vi "Session.vi"() -> ()   [LabVIEW 2017]
uses:
  Control/Damping.ctl
  Global.vi
panel:
  in  "Type":enum16{"Mini45", "Joystick", "Simulation"}(ring)=enum."Simulation"
  out "Waveform Chart":dbl(graph)
  out "Reward":dbl(graph)
  out "Damping":T1={"Cx"=0.5493061443340549, "Cy"=0.5493061443340549, "Cz"=inf}
  in  "DDA":bool=TRUE
  out "error out":errorcluster
  in  "Stop":bool
  in  "error in":errorcluster
  in  "Exit":bool
  in  "Start":bool
  in  "ADL":u16(ring)=2 items=["None", "Book", "Pitcher", "Laptop", "Gear"]
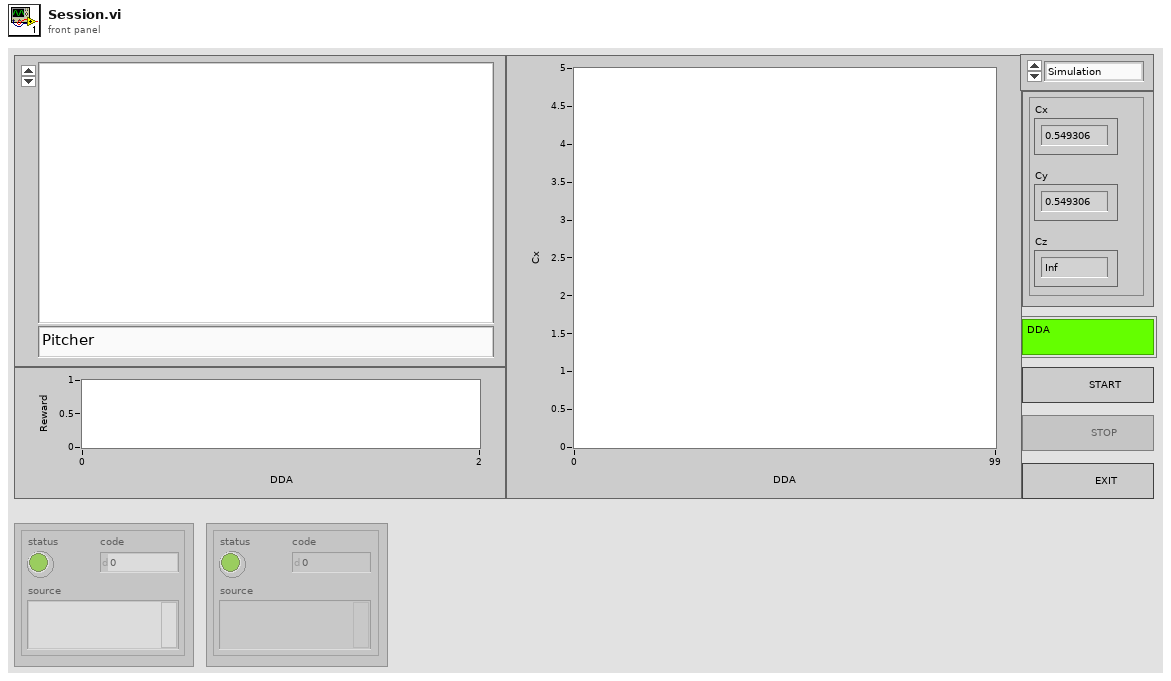
[diagram p1: front panel]
types:
  T1 = typedef "Damping.ctl" = cluster{"Cx":dbl, "Cy":dbl, "Cz":dbl}
  T2 = enum8{"Enabled", "Disabled", "Disabled and Grayed Out"}
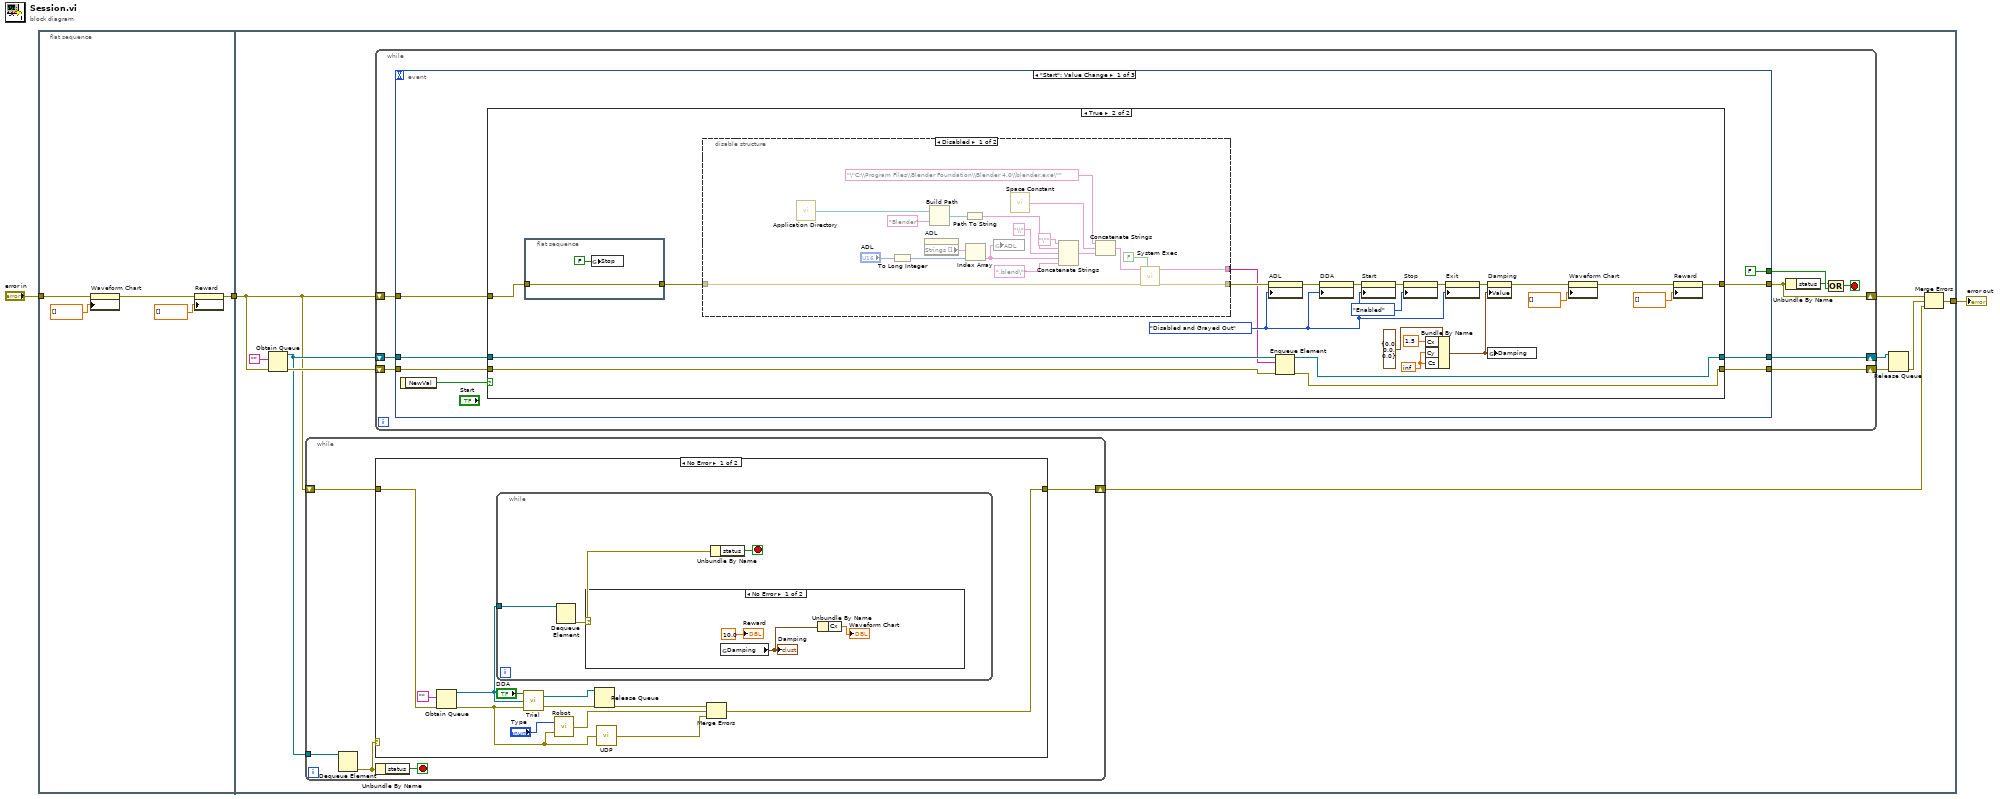
[diagram p0: block diagram]
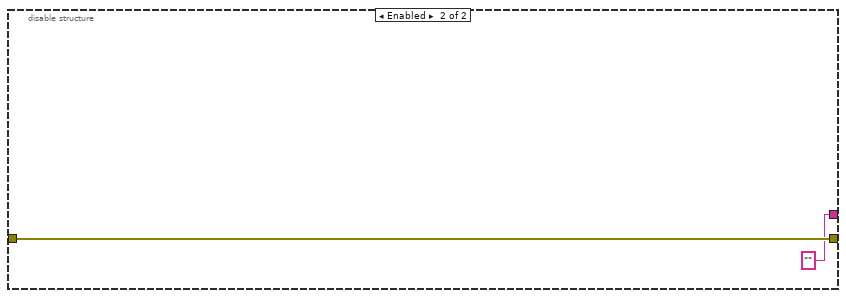
[diagram p3: hidden frame]
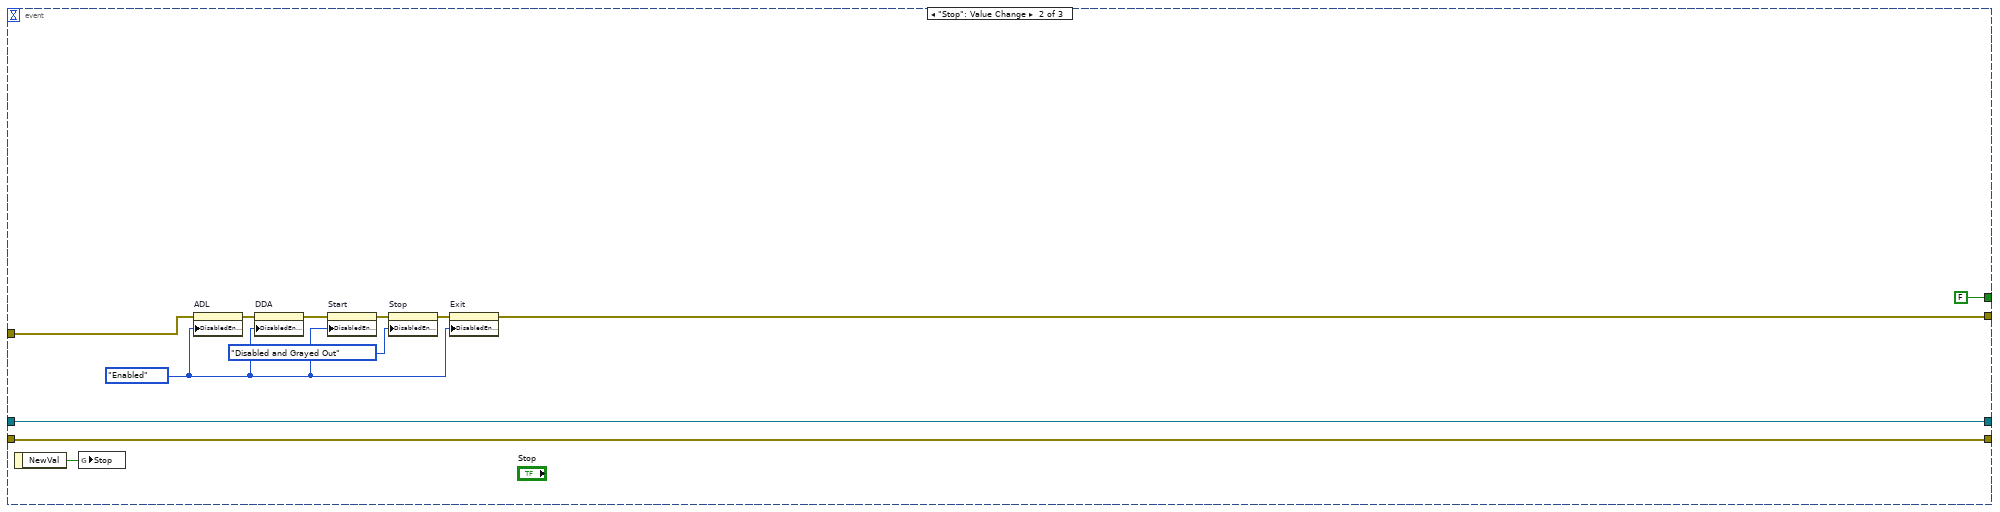
[diagram p4: hidden frame]
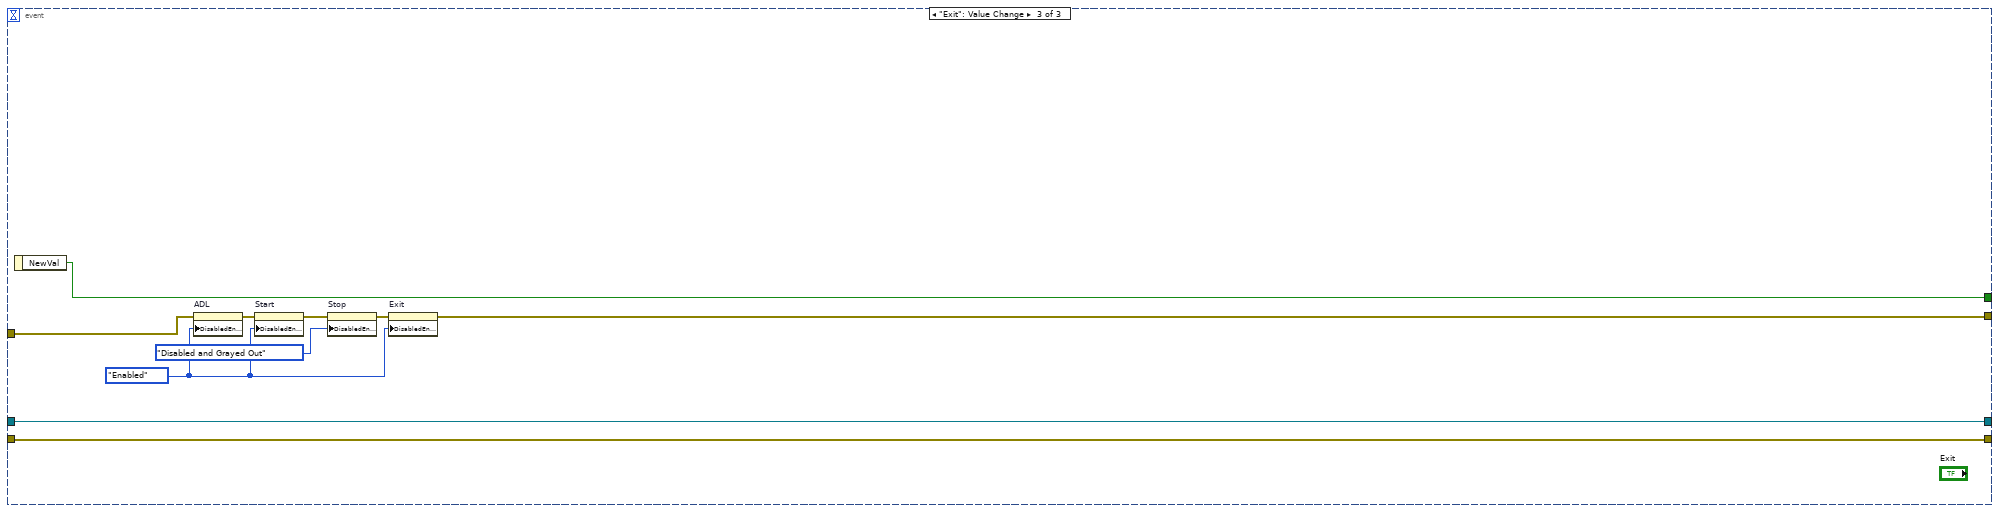
[diagram p5: hidden frame]
diagram:
  n1 = flat-sequence {
    tunnel: "error in" -> [w6]
    tunnel: [w4] -> w1
    tunnel: [w11] -> w3
    tunnel: w1 -> [w9]
    frame #0 {
      n2 = property on="Waveform Chart" class="WFChart (strict)"(error in=w6, "History Data"=dbl[] []) -> (error out=w5:errorcluster)  [unwired: 1 in, 1 out]
      n3 = property on="Reward" class="WFChart (strict)"(error in=w5, "History Data"=dbl[] []) -> (error out=w4:errorcluster)  [unwired: 1 in, 1 out]
    }
    frame #1 {
      n4 = Obtain Queue(element data type="", error in (no error)=w9) -> (queue out=w14:refnum<queue>, error out=w17:errorcluster)  [unwired: 3 in, 1 out]
      n5 = while {
        tunnel: w14 -> [w112]
        shift-right: [w109] -> w10
        shift-left: w9 -> [w108]
        stop <- w110 stop-if-true
        n6 = Dequeue Element(queue=w112) -> (error out=w111:errorcluster)  [unwired: 2 in, 3 out]
        n7 = case shown="No Error" w111 {
          tunnel: [w123 w131] -> w109
          tunnel: w108 -> [w122 w131]
          frame No Error {
            n8 = Obtain Queue(element data type="", error in (no error)=w122) -> (queue out=w116:refnum<queue>, error out=w115:errorcluster)  [unwired: 3 in, 1 out]
            n9 = while {
              tunnel: w116 -> [w126]
              stop <- w125 stop-if-true
              n10 = Dequeue Element(queue=w126) -> (error out=w127:errorcluster)  [unwired: 2 in, 3 out]
              n11 = case shown="No Error" w127 {
                frame No Error {
                  n12 = global read "Global.vi" "Damping"() -> (w130:T1)
                  "Damping" <- w130
                  n13 = Unbundle By Name(w130) -> ("Cx"=→"Waveform Chart":dbl)
                  "Reward" <- 10.0 ("Reward")
                }
                frame Error {
                }
              }
              n14 = Unbundle By Name(w127) -> ("status"=w125:bool)
            }
            n15 = call "Trial.vi"("error in (no error)"=w115, "queue in"=w116, "DDA"="DDA") -> ("error out"=w114:errorcluster, "queue out"=w113:refnum<queue>)
            n16 = call "Robot.vi"("error in"=w115, "Type"="Type") -> ("error out"=w119:errorcluster)
            n17 = Release Queue(queue=w113, error in (no error)=w114) -> (error out=w120:errorcluster)  [unwired: 1 in, 2 out]
            n18 = call "UDP.vi"("error in (no error)"=w115) -> ("error out"=w124:errorcluster)
            n19 = Merge Errors(w120, w119, w124) -> (w123:errorcluster)
          }
          frame Error {
          }
        }
        n20 = Unbundle By Name(w111) -> ("status"=w110:bool)
      }
      n21 = while {
        shift-right: [w26] -> w13
        shift-left: w9 -> [w27]
        shift-right: [w19] -> w15
        shift-left: w17 -> [w21]
        shift-right: [w20] -> w16
        shift-left: w14 -> [w22]
        stop <- w23 stop-if-true
        n22 = event shown="[0] \"Start\": Value Change" {
          selector: _ -> [_ _ _]
          dyn-events: _ -> [_ _ _]
          timeout: _ -> [_ _ _]
          tunnel: [w34 w93 w100] -> w26
          tunnel: w27 -> [w33 w86 w104]
          tunnel: [FALSE ("Stop") FALSE ("NewVal") w107] -> w25
          tunnel: w22 -> [w31 w94 w106]
          tunnel: w21 -> [w30 w95 w105]
          tunnel: [w29 w94 w106] -> w20
          tunnel: [w28 w95 w105] -> w19
          event "Start": Value Change {
            n23 = event-data() -> ("NewVal"=w35:bool)  [unwired: 1 in]
            n24 = case shown="True" w35 {
              tunnel: [w38 w45] -> w34
              tunnel: w33 -> [w38 w51]
              tunnel: w31 -> [w36 w62]
              tunnel: w30 -> [w37 w61]
              tunnel: [w36 w60] -> w29
              tunnel: [w37 w59] -> w28
              frame False {
              }
              frame True {
                w39 = inf
                w53 = T2."Disabled and Grayed Out" ("Disabled")
                n25 = flat-sequence {
                  tunnel: [w84] -> w49
                  tunnel: w51 -> [w84]
                  frame #0 {
                    n26 = global write "Global.vi" "Stop"(FALSE ("Stop")) -> ()
                  }
                }
                n27 = disable-structure shown="Disabled" {
                  disable-tunnel: [w69 w83] -> w58
                  disable-tunnel: w49 -> [w64 w83]
                  disable-tunnel: [w63 "" ("standard output")] -> w41
                  frame Disabled {
                    n28 = call <vilib>:"Application Directory.vi"() -> ("Application Directory"=w79:path)
                    n29 = To Long Integer(number="ADL") -> (32bit integer=w68:i32)
                    n30 = property on="ADL" class="Ring (strict)"() -> ("Strings []"=w81:string[])  [unwired: 2 in, 2 out]
                    n31 = Build Path(base path=w79, name or relative path="Blender") -> (appended path=w77:path)
                    n32 = Path To String(path=w77) -> (string=w76:string)
                    n33 = Index Array(array=w81, index=w68) -> (element=w67:string)
                    n34 = global write "Global.vi" "ADL"(w67) -> ()
                    n35 = call <vilib>:"Space Constant.vi"() -> ("String"=w72:string)
                    n36 = Concatenate Strings("\"" ("string"), w76, "\\" ("string"), w67, ".blend\"" ("string")) -> (w71:string)
                    n37 = Concatenate Strings("\"C:\\Program Files\\Blender Foundation\\Blender 4.0\\blender.exe\"" ("Blender Path"), w72, w71) -> (w70:string)
                    n38 = call <vilib>:"System Exec.vi"("wait until completion? (T)"=FALSE, "error in (no error)"=w64, "command line"=w70) -> ("error out"=w69:errorcluster, "standard output"=w63:string)  [unwired: 5 in, 2 out]
                  }
                  frame Enabled {
                  }
                }
                n39 = property on="ADL" class="Ring (strict)"(error in=w58, "DisabledEnum"=w53) -> (error out=w52:errorcluster)  [unwired: 1 in, 1 out]
                n40 = Enqueue Element(queue=w62, element=w41, error in (no error)=w61) -> (queue out=w60:refnum<queue>, error out=w59:errorcluster)  [unwired: 1 in, 1 out]
                n41 = property on="DDA" class="Bool (strict)"(error in=w52, "DisabledEnum"=w53) -> (error out=w54:errorcluster)  [unwired: 1 in, 1 out]
                n42 = property on="Start" class="Bool"(error in=w54, "DisabledEnum"=w53) -> (error out=w57:errorcluster)  [unwired: 1 in, 1 out]
                n43 = property on="Stop" class="Bool"(error in=w57, "DisabledEnum"=T2."Enabled" ("Disabled")) -> (error out=w56:errorcluster)  [unwired: 1 in, 1 out]
                n44 = Bundle By Name(cluster=T1 {"Cx"=0.0, "Cy"=0.0, "Cz"=0.0} ("State"), "Cx"=1.5, "Cy"=w39, "Cz"=w39) -> (w48:T1)
                n45 = property on="Exit" class="Bool"(error in=w56, "DisabledEnum"=w53) -> (error out=w47:errorcluster)  [unwired: 1 in, 1 out]
                n46 = property on="Damping" class="Clust (strict)"(error in=w47, "Value"=w48) -> (error out=w44:errorcluster)  [unwired: 1 in, 1 out]
                n47 = global write "Global.vi" "Damping"(w48) -> ()
                n48 = property on="Waveform Chart" class="WFChart (strict)"(error in=w44, "History Data"=dbl[] []) -> (error out=w43:errorcluster)  [unwired: 1 in, 1 out]
                n49 = property on="Reward" class="WFChart (strict)"(error in=w43, "History Data"=dbl[] []) -> (error out=w45:errorcluster)  [unwired: 1 in, 1 out]
              }
            }
          }
          event "Stop": Value Change {
            w87 = T2."Enabled" ("Disabled")
            n50 = event-data() -> ("NewVal"=w97:bool)  [unwired: 1 in]
            n51 = global write "Global.vi" "Stop"(w97) -> ()
            n52 = property on="ADL" class="Ring (strict)"(error in=w86, "DisabledEnum"=w87) -> (error out=w89:errorcluster)  [unwired: 1 in, 1 out]
            n53 = property on="DDA" class="Bool (strict)"(error in=w89, "DisabledEnum"=w87) -> (error out=w88:errorcluster)  [unwired: 1 in, 1 out]
            n54 = property on="Start" class="Bool"(error in=w88, "DisabledEnum"=w87) -> (error out=w92:errorcluster)  [unwired: 1 in, 1 out]
            n55 = property on="Stop" class="Bool"(error in=w92, "DisabledEnum"=T2."Disabled and Grayed Out" ("Disabled")) -> (error out=w91:errorcluster)  [unwired: 1 in, 1 out]
            n56 = property on="Exit" class="Bool"(error in=w91, "DisabledEnum"=w87) -> (error out=w93:errorcluster)  [unwired: 1 in, 1 out]
          }
          event "Exit": Value Change {
            w99 = T2."Enabled" ("Disabled")
            n57 = event-data() -> ("NewVal"=w107:bool)  [unwired: 1 in]
            n58 = property on="ADL" class="Ring (strict)"(error in=w104, "DisabledEnum"=w99) -> (error out=w101:errorcluster)  [unwired: 1 in, 1 out]
            n59 = property on="Start" class="Bool"(error in=w101, "DisabledEnum"=w99) -> (error out=w103:errorcluster)  [unwired: 1 in, 1 out]
            n60 = property on="Stop" class="Bool"(error in=w103, "DisabledEnum"=T2."Disabled and Grayed Out" ("Disabled")) -> (error out=w102:errorcluster)  [unwired: 1 in, 1 out]
            n61 = property on="Exit" class="Bool"(error in=w102, "DisabledEnum"=w99) -> (error out=w100:errorcluster)  [unwired: 1 in, 1 out]
          }
        }
        n62 = Unbundle By Name(w26) -> ("status"=w24:bool)
        n63 = Compound Arithmetic op=OR(w24, w25) -> (w23:bool)
      }
      n64 = Release Queue(queue=w16, error in (no error)=w15) -> (error out=w12:errorcluster)  [unwired: 1 in, 2 out]
      n65 = Merge Errors(w13, w12, w10) -> (w11:errorcluster)
    }
  }
  "error out" <- w3
